vi "_Parse Limit Check Array Result.vi"(0 "error in (no error)":errorcluster, 2 "Input String":string, 3 "VISA resource name":refnum<visa-resource-name>, 4 "Out of tolerance? (F)":bool) -> (7 "error out":errorcluster, 8 "Results":i32[](array[numeric]), 9 "Reliability":i32, 10 "VISA resource name out":refnum<visa-resource-name>)   [LabVIEW 2020, in "Rohde&Schwarz CMXP NR FR2 Measurement.lvlib"]
uses:
  <instrlib>/Rohde&Schwarz CMXP NR FR2 Measurement/Rohde&Schwarz CMXP NR FR2 Measurement.lvlib
  <instrlib>/Rohde&Schwarz CMXP NR FR2 Measurement/Private/rsidr_core.llb/rsidr_core.lvlib
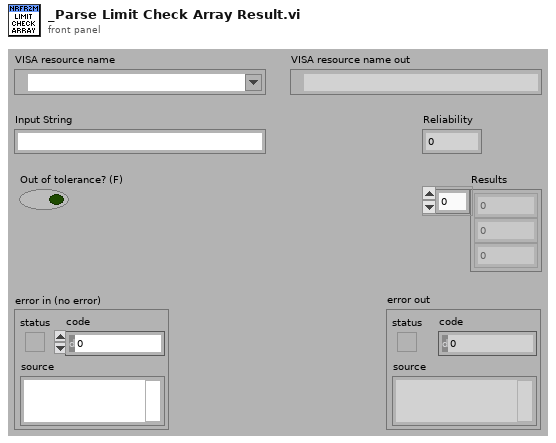
[diagram p1: front panel]
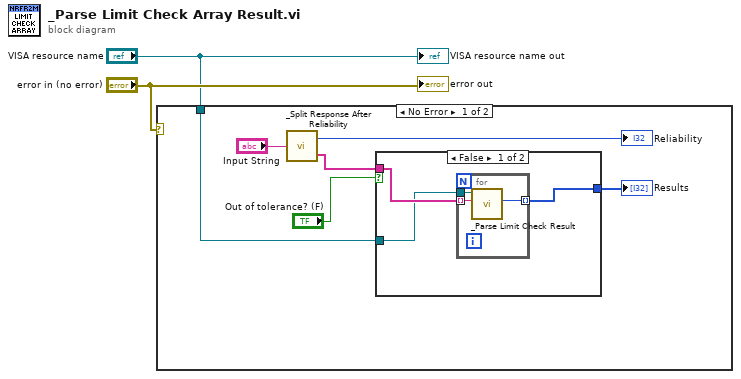
[diagram p0: block diagram]
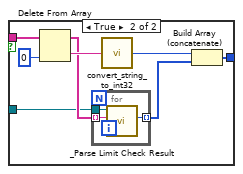
[diagram p2: hidden frame]
diagram:
  n1 = case shown="No Error" "error in (no error)" {
    tunnel: "VISA resource name" -> [w3 _]
    frame No Error {
      n2 = call <instrlib>:"_Split Response After Reliability.vi"("Input String"="Input String") -> ("Response out"=w6:string[], "Reliability out"=→"Reliability":i32)
      n3 = case shown="False" "Out of tolerance? (F)" {
        tunnel: w6 -> [w11 w22]
        tunnel: [w10 w18] -> w5
        tunnel: w3 -> [w9 w15]
        frame False {
          n4 = for {
            tunnel: [w14] -> w10 mode=indexing
            tunnel: w11 -> [w13] mode=indexing
            tunnel: w9 -> [w12]
            n5 = call <instrlib>:"_Parse Limit Check Result.vi"("String Value In"=w13, "VISA resource name"=w12) -> ("Limit Check Value"=w14:i32)  [unwired: 7 in, 2 out]
          }
        }
        frame True {
          n6 = Delete From Array(array=w22, index=0) -> (deleted portion=w20:string, array with subset deleted=w17:string[])  [unwired: 1 in]
          n7 = for {
            tunnel: [w25] -> w16 mode=indexing
            tunnel: w17 -> [w24] mode=indexing
            tunnel: w15 -> [w23]
            n8 = call <instrlib>:"_Parse Limit Check Result.vi"("String Value In"=w24, "VISA resource name"=w23) -> ("Limit Check Value"=w25:i32)  [unwired: 7 in, 2 out]
          }
          n9 = call <instrlib>:"convert_string_to_int32.vi"("String in"=w20) -> ("int32 value out"=w19:i32)  [unwired: 4 in]
          n10 = Build Array (concatenate)(w19, w16) -> (w18:i32[])
        }
      }
      "Results" <- w5
    }
    frame Error {
    }
  }
  "VISA resource name out" <- "VISA resource name"
  "error out" <- "error in (no error)"
